vi "add tag sub.vi"(5 "Class":bool=TRUE, 6 "index":i32, 7 "sort Enum":enum16{"CName", "CNO", "ClassI", "ClassII"}(ring), 8 "error in (no error)":errorcluster, 9 "Parent Tag":string, 10 "CH_sort in":T1[](array[typedef]) {"CHS"."display" format="%b"}, 11 "reference":refnum<vi>) -> (0 "error out":errorcluster, 1 "child tag":string, 2 "CH_sort":T1[](array[typedef]) {"CHS"."display" format="%b"}, 3 "reference out":refnum<vi>, 4 "stop?":bool)   [LabVIEW 2011]
uses:
  chs_sort.ctl
  CHS.ctl
  singlechtype.ctl
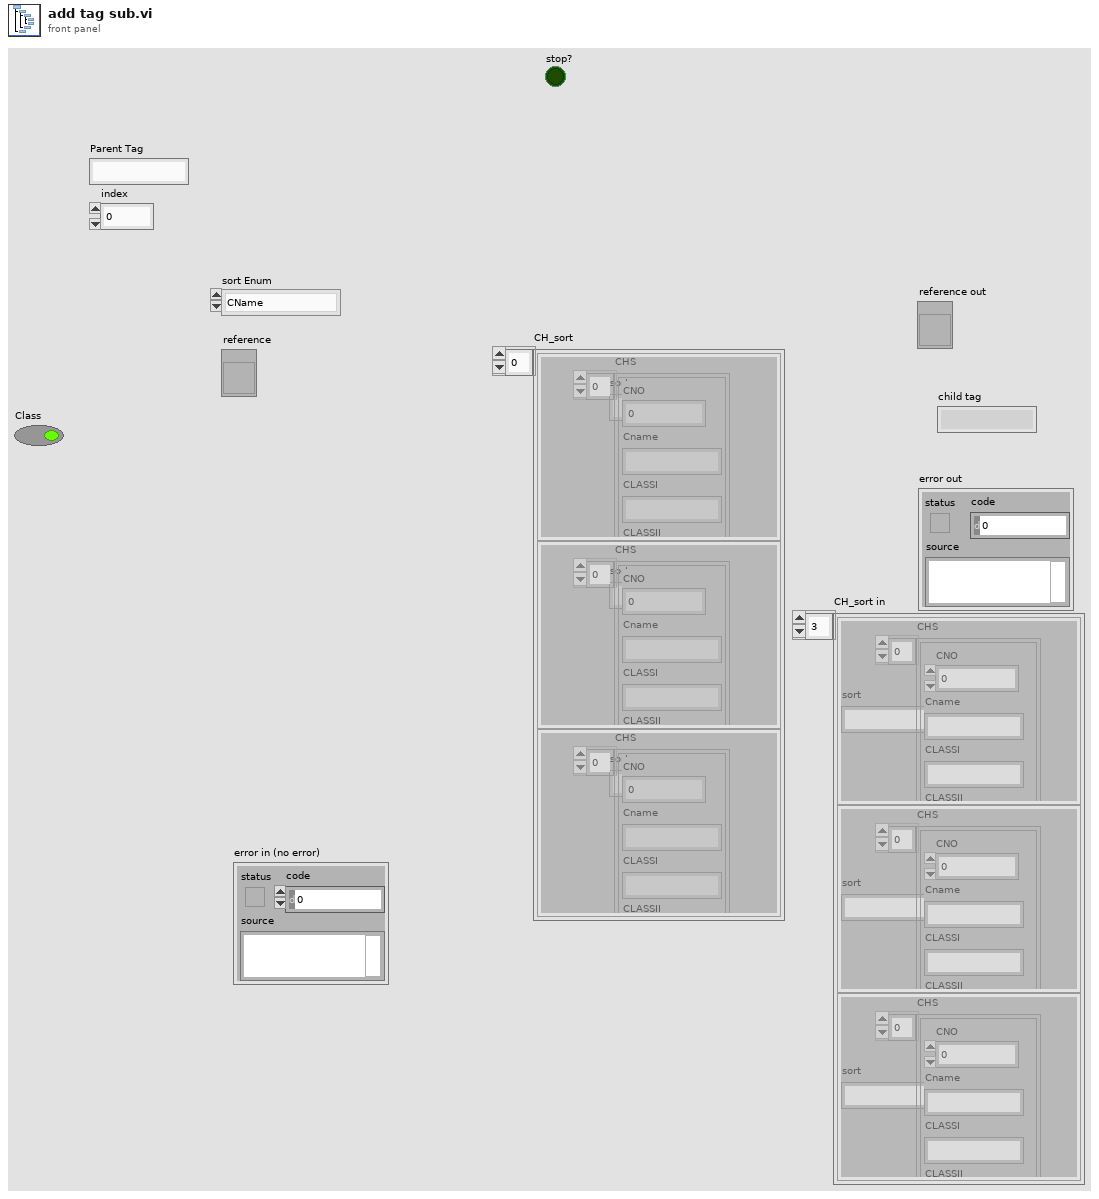
[diagram p1: front panel]
types:
  T1 = typedef "chs_sort.ctl" = cluster{"sort":string, "CHS":T2}
  T2 = typedef "CHS.ctl" = T3[]
  T3 = typedef "singlechtype.ctl" = cluster{"CNO":u8, "Cname":string, "CLASSI":string, "CLASSII":string, "Ch":u8, "CHName":string, "USE":bool, "fre":dbl, "range":enum16{""}, "SenNO":string, "PHname":string, "unit":string, "CALClass":enum8{"线性", "查表", "公式"}, "K":dbl, "OFF":dbl, "Alrm":bool, "Filt":dbl, "Power":u8, "display":u8, "threshold ":dbl, "Enum":enum16{">", ">=", "<", "<=", "<>(在范围内）", "><（在范围外）"}, "Etype":enum16{"电压", "电流", "电阻", "热电偶K", "热电偶T"}}
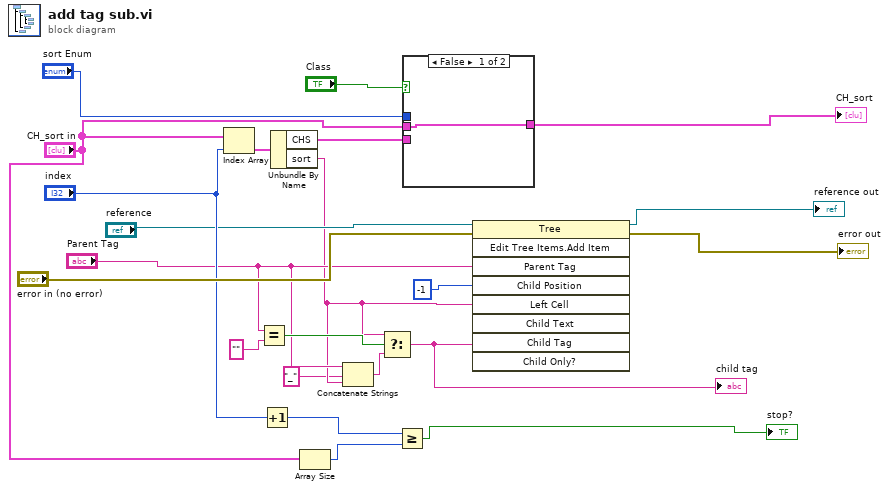
[diagram p0: block diagram]
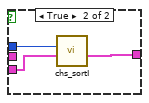
[diagram p2: hidden frame]
diagram:
  n1 = Index Array(array="CH_sort in", index="index") -> (element=w12:T1)
  n2 = Equal?(x="Parent Tag", y="" ("Parent Tag")) -> (x = y?=w9:bool)
  n3 = Increment(x="index") -> (x+1=w10:i32)
  n4 = Unbundle By Name(w12) -> ("CHS"=w14:T2, "sort"=w5:string)
  n5 = Array Size(array="CH_sort in") -> (size(s)=w11:i32)
  n6 = Concatenate Strings("Parent Tag", "_" ("string"), w5) -> (w7:string)
  n7 = Select(t=w5, s=w9, f=w7) -> (s? t:f=w6:string)
  "child tag" <- w6
  n8 = Greater Or Equal?(x=w10, y=w11) -> (x >= y?=→"stop?":bool)
  n9 = case shown="False" "Class" {
    tunnel: [w23 w26] -> w22
    tunnel: "sort Enum" -> [_ w25]
    tunnel: w14 -> [_ w24]
    tunnel: "CH_sort in" -> [w23 _]
    frame False {
    }
    frame True {
      n10 = call "chs_sortI.vi"("CHS"=w24, "Enum"=w25) -> ("CH_sort"=w26:T1[])  [unwired: 9 in]
    }
  }
  "CH_sort" <- w22
  n11 = invoke class="Tree" method="Edit Tree Items.Add Item"(reference="reference", error in="error in (no error)", "Parent Tag"="Parent Tag", "Child Position"=-1, "Left Cell"=w5, "Child Tag"=w6) -> (reference out=→"reference out":refnum<vi>, error out=→"error out":errorcluster)  [unwired: 3 in, 7 out]
